vi "Prober_ThetaAlignment.vi"(4 "y2":i32, 5 "y1":i32, 6 "x2":i32, 7 "x1":i32, 8 "error in (no error)":errorcluster, 11 "SemiProbe in":refnum<class "SemiProbe.lvclass">) -> (0 "error out":errorcluster, 1 "theta increment":i32, 2 "New millidegrees":i32, 3 "SemiProbe out":refnum<class "SemiProbe.lvclass">)   [LabVIEW 2013, in "SemiProbe.lvclass"]
uses:
  SemiProbe.lvclass
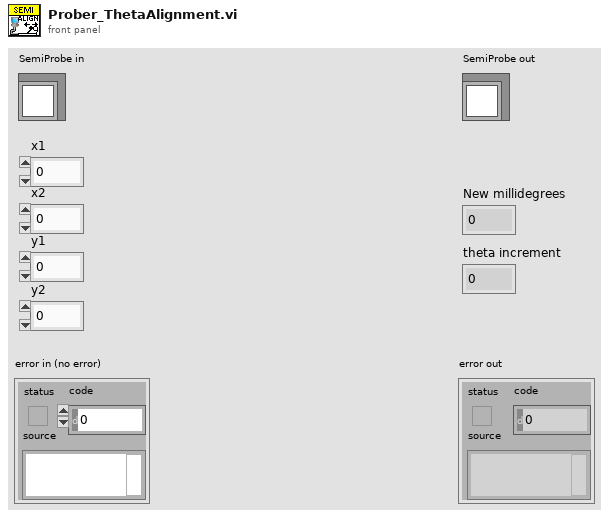
[diagram p1: front panel]
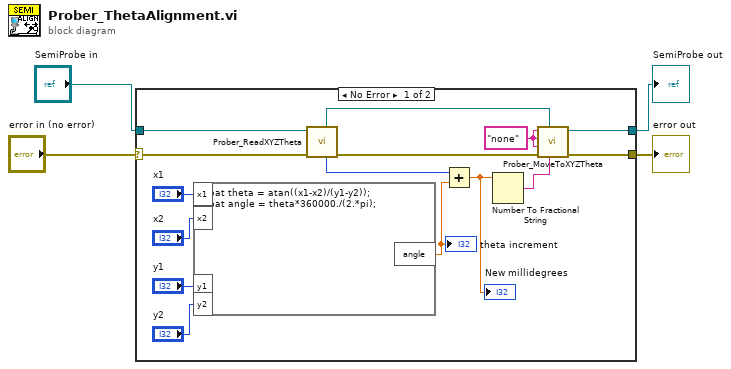
[diagram p0: block diagram]
diagram:
  n1 = case shown="No Error" "error in (no error)" {
    selector: "error in (no error)" -> [w11 w20]
    tunnel: "SemiProbe in" -> [w14 w21]
    tunnel: [w13 w21] -> w3
    tunnel: [w12 w20] -> w2
    frame No Error {
      w10 = "none"
      n2 = formula code="float theta = atan((x1-x2)/(y1-y2));\nfloat angle = theta*360000./(2.*pi);"("x1"="x1", "x2"="x2", "y1"="y1", "y2"="y2") -> ("angle"=w7:dbl)
      "theta increment" <- w7
      n3 = call-dynamic "Prober_ReadXYZTheta.vi"("error in (no error)"=w11, "SemiProbe in"=w14) -> ("error out"=w9:errorcluster, "Theta location [mdeg]"=w6:i32, "SemiProbe out"=w15:refnum<class "SemiProbe.lvclass">)  [unwired: 4 in, 3 out]
      n4 = Add(x=w6, y=w7) -> (x+y=w5:dbl)
      "New millidegrees" <- w5
      n5 = Number To Fractional String(number=w5) -> (F-format string=w8:string)  [unwired: 3 in]
      n6 = call-dynamic "Prober_MoveToXYZTheta.vi"("Theta location [mdeg]"=w8, "SemiProbe in"=w15, "error in (no error)"=w9, "Z location [µm]"=w10, "Y location [µm]"=w10, "X location [µm]"=w10) -> ("error out"=w12:errorcluster, "SemiProbe out"=w13:refnum<class "SemiProbe.lvclass">)  [unwired: 3 in, 1 out]
    }
    frame Error {
    }
  }
  "error out" <- w2
  "SemiProbe out" <- w3
